vi "TrajectoryParam_calcStuffFwd.vi"(4 "TRAJECTORY_CONFIG":T1={"MaxVelocity"=0.0, "Max Acceleration"=0.0, "StartVelocity"=0.0, "End Velocity"=0.0, "Reversed"=FALSE, "DiffDrKineConstntDefined"=FALSE, "CentAcellConstntDefined"=FALSE, "DiffDrVoltConstntDefined"=FALSE, "DIFF_DRIVE_KINE_CONSTRAINT"={"Max Speed (M/S)"=0.0, "DIFF_DRIVE_KINEMATICS"={"TrackWidth_Meters"=0.0}}, "CENTRIPETAL_ACCEL_CONSTRAINT"={"Max Cent Accel"=0.0}, "SwerveDrKineConstntDefined"=FALSE, "SWERVE_DRIVE_KINE_CONSTRAINT"={"Max Speed (M/S)"=0.0, "SwerveKinematics"={"NumModules"=0, "InverseKinematics"=[], "ForwardKinematics"=[], "Modules"=[], "PrevCoR"={"X"=0.0, "Y"=0.0}}}, "DIFF_DRIVE_VOLTAGE_CONSTRAINT"={"Max Voltage"=0.0, "DIFF_DRIVE_KINEMATICS"={"TrackWidth_Meters"=0.0}, "SIMPLE_MOTOR_FF"={"Ks"=0.0, "Kv"=0.0, "Ka"=0.0}}, "MECANUM_DRIVE_KINE_CONSTRAINT"={"Max Speed (M/S)"=0.0, "MECA_DRIVE_KINEMATICS"={"FrontLeft"={"X"=0.0, "Y"=0.0}, "FrontRight"={"X"=0.0, "Y"=0.0}, "RearLeft"={"X"=0.0, "Y"=0.0}, "RearRight"={"X"=0.0, "Y"=0.0}, "InverseKinematics"=[[0.0, 1.0, -1.0, 0.0], [0.0, 1.0, 1.0, 0.0], [0.0, 1.0, 1.0, 0.0], [0.0, 1.0, -1.0, 0.0]], "ForwardKinematics"=[[0.0, 1.0, -1.0, 0.0], [0.0, 1.0, 1.0, 0.0], [0.0, 1.0, 1.0, 0.0], [0.0, 1.0, -1.0, 0.0]], "PrevCoR"={"X"=0.0, "Y"=0.0}}}, "MecanumDrKineConstntDefined"=FALSE} {"MECANUM_DRIVE_KINE_CONSTRAINT"."MECA_DRIVE_KINEMATICS"."PrevCoR"."Y" format="%14.3f"; "MECANUM_DRIVE_KINE_CONSTRAINT"."MECA_DRIVE_KINEMATICS"."PrevCoR"."X" format="%14.3f"; "MECANUM_DRIVE_KINE_CONSTRAINT"."MECA_DRIVE_KINEMATICS"."RearRight"."Y" format="%14.3f"; "MECANUM_DRIVE_KINE_CONSTRAINT"."MECA_DRIVE_KINEMATICS"."RearRight"."X" format="%14.3f"; "MECANUM_DRIVE_KINE_CONSTRAINT"."MECA_DRIVE_KINEMATICS"."RearLeft"."Y" format="%14.3f"; "MECANUM_DRIVE_KINE_CONSTRAINT"."MECA_DRIVE_KINEMATICS"."RearLeft"."X" format="%14.3f"; "MECANUM_DRIVE_KINE_CONSTRAINT"."MECA_DRIVE_KINEMATICS"."FrontRight"."Y" format="%14.3f"; "MECANUM_DRIVE_KINE_CONSTRAINT"."MECA_DRIVE_KINEMATICS"."FrontRight"."X" format="%14.3f"; "MECANUM_DRIVE_KINE_CONSTRAINT"."MECA_DRIVE_KINEMATICS"."FrontLeft"."Y" format="%14.3f"; "MECANUM_DRIVE_KINE_CONSTRAINT"."MECA_DRIVE_KINEMATICS"."FrontLeft"."X" format="%14.3f"; "MECANUM_DRIVE_KINE_CONSTRAINT"."Max Speed (M/S)" format="%20.4f"; "DIFF_DRIVE_VOLTAGE_CONSTRAINT"."SIMPLE_MOTOR_FF"."Ka" format="%13.4f"; "DIFF_DRIVE_VOLTAGE_CONSTRAINT"."SIMPLE_MOTOR_FF"."Kv" format="%13.4f"; "DIFF_DRIVE_VOLTAGE_CONSTRAINT"."SIMPLE_MOTOR_FF"."Ks" format="%13.4f"; "DIFF_DRIVE_VOLTAGE_CONSTRAINT"."DIFF_DRIVE_KINEMATICS"."TrackWidth_Meters" format="%20.4f"; "DIFF_DRIVE_VOLTAGE_CONSTRAINT"."Max Voltage" format="%20.4f"; "SWERVE_DRIVE_KINE_CONSTRAINT"."SwerveKinematics"."PrevCoR"."Y" format="%14.3f"; "SWERVE_DRIVE_KINE_CONSTRAINT"."SwerveKinematics"."PrevCoR"."X" format="%14.3f"; "SWERVE_DRIVE_KINE_CONSTRAINT"."SwerveKinematics"."Modules"."Y" format="%14.3f"; "SWERVE_DRIVE_KINE_CONSTRAINT"."SwerveKinematics"."Modules"."X" format="%14.3f"; "SWERVE_DRIVE_KINE_CONSTRAINT"."Max Speed (M/S)" format="%20.4f"; "CENTRIPETAL_ACCEL_CONSTRAINT"."Max Cent Accel" format="%20.4f"; "DIFF_DRIVE_KINE_CONSTRAINT"."DIFF_DRIVE_KINEMATICS"."TrackWidth_Meters" format="%20.4f"; "DIFF_DRIVE_KINE_CONSTRAINT"."Max Speed (M/S)" format="%20.4f"; "End Velocity" format="%20.4f"; "StartVelocity" format="%20.4f"; "Max Acceleration" format="%20.4f"; "MaxVelocity" format="%20.4f"}, 6 "MaxVelocity":dbl, 7 "Reversed":bool, 8 "MaxAccel":dbl, 9 "previousCONSTRAINED_STATEin":T13={"POSEwCURVATURE"={"CURVATURE"=0.0, "POSE"={"TRANSLATION"={"X"=0.0, "Y"=0.0}, "ROTATION"={"VALUE"=0.0, "COS"=1.0, "SIN"=0.0}}}, "Distance"=0.0, "minAccel"=0.0, "maxAccel"=0.0, "maxVelocity"=0.0} {"POSEwCURVATURE"."POSE"."ROTATION"."SIN" format="%13.4f"; "POSEwCURVATURE"."POSE"."ROTATION"."COS" format="%13.4f"; "POSEwCURVATURE"."POSE"."ROTATION"."VALUE" format="%13.4f"; "POSEwCURVATURE"."POSE"."TRANSLATION"."Y" format="%14.3f"; "POSEwCURVATURE"."POSE"."TRANSLATION"."X" format="%14.3f"}, 10 "ds":dbl, 11 "thisCONSTRAINED_STATEin":T13={"POSEwCURVATURE"={"CURVATURE"=0.0, "POSE"={"TRANSLATION"={"X"=0.0, "Y"=0.0}, "ROTATION"={"VALUE"=0.0, "COS"=1.0, "SIN"=0.0}}}, "Distance"=0.0, "minAccel"=0.0, "maxAccel"=0.0, "maxVelocity"=0.0} {"POSEwCURVATURE"."POSE"."ROTATION"."SIN" format="%13.4f"; "POSEwCURVATURE"."POSE"."ROTATION"."COS" format="%13.4f"; "POSEwCURVATURE"."POSE"."ROTATION"."VALUE" format="%13.4f"; "POSEwCURVATURE"."POSE"."TRANSLATION"."Y" format="%14.3f"; "POSEwCURVATURE"."POSE"."TRANSLATION"."X" format="%14.3f"}) -> (0 "error out":errorcluster, 1 "previousCONSTRAINED_STATEout":T13={"POSEwCURVATURE"={"CURVATURE"=0.0, "POSE"={"TRANSLATION"={"X"=0.0, "Y"=0.0}, "ROTATION"={"VALUE"=0.0, "COS"=1.0, "SIN"=0.0}}}, "Distance"=0.0, "minAccel"=0.0, "maxAccel"=0.0, "maxVelocity"=0.0} {"POSEwCURVATURE"."POSE"."ROTATION"."SIN" format="%13.4f"; "POSEwCURVATURE"."POSE"."ROTATION"."COS" format="%13.4f"; "POSEwCURVATURE"."POSE"."ROTATION"."VALUE" format="%13.4f"; "POSEwCURVATURE"."POSE"."TRANSLATION"."Y" format="%14.3f"; "POSEwCURVATURE"."POSE"."TRANSLATION"."X" format="%14.3f"}, 3 "thisCONSTRAINED_STATEout":T13={"POSEwCURVATURE"={"CURVATURE"=0.0, "POSE"={"TRANSLATION"={"X"=0.0, "Y"=0.0}, "ROTATION"={"VALUE"=0.0, "COS"=1.0, "SIN"=0.0}}}, "Distance"=0.0, "minAccel"=0.0, "maxAccel"=0.0, "maxVelocity"=0.0} {"POSEwCURVATURE"."POSE"."ROTATION"."SIN" format="%13.4f"; "POSEwCURVATURE"."POSE"."ROTATION"."COS" format="%13.4f"; "POSEwCURVATURE"."POSE"."ROTATION"."VALUE" format="%13.4f"; "POSEwCURVATURE"."POSE"."TRANSLATION"."Y" format="%14.3f"; "POSEwCURVATURE"."POSE"."TRANSLATION"."X" format="%14.3f"})   [LabVIEW 2019, in "Trajectory_Library.lvlib"]
doc: "Internal routine called by TrajectoryParam_timeParam.VI"
uses:
  Trajectory_Library.lvlib
  CONSTRAINED_STATE.ctl
  POSEwCURVATURE.ctl
  POSE2D.ctl
  TRANSLATION2D.ctl
  ROTATION2D.ctl
  TRAJ_CONFIG.ctl
  TRAJ_CONSTRAINT_DIIF_DRIVE_KINEMATICS.ctl
  DIFF_DRIVE_KINEMATICS.ctl
  TRAJ_CONSTRAINT_CENTRIPETAL_ACCEL.ctl
  TRAJ_CONSTRAINT_SWERVE_DRIVE_KINEMATICS.ctl
  SWERVE_DRIVE_KINEMATICS.ctl
  <vilib>/Analysis/Matrix/Datatypes/RealMatrix.ctl
  TRAJ_CONSTRAINT_DIIF_DRIVE_VOLTAGE.ctl
  SIMPLE_MOTOR_FF.ctl
  TRAJ_CONSTRAINT_MECA_DRIVE_KINEMATICS.ctl
  MECA_DRIVE_KINEMATICS.ctl
  <vilib>/Analysis/Matrix/NI_Matrix.lvlib
panel:
  # "ARRAY OF OTHER\nCONSTRAINTS \nGOES HERE.."
  # "All units\nare SI"
  # "All units\nare SI"
  # "All units\nare SI"
  # "All units\nare SI"
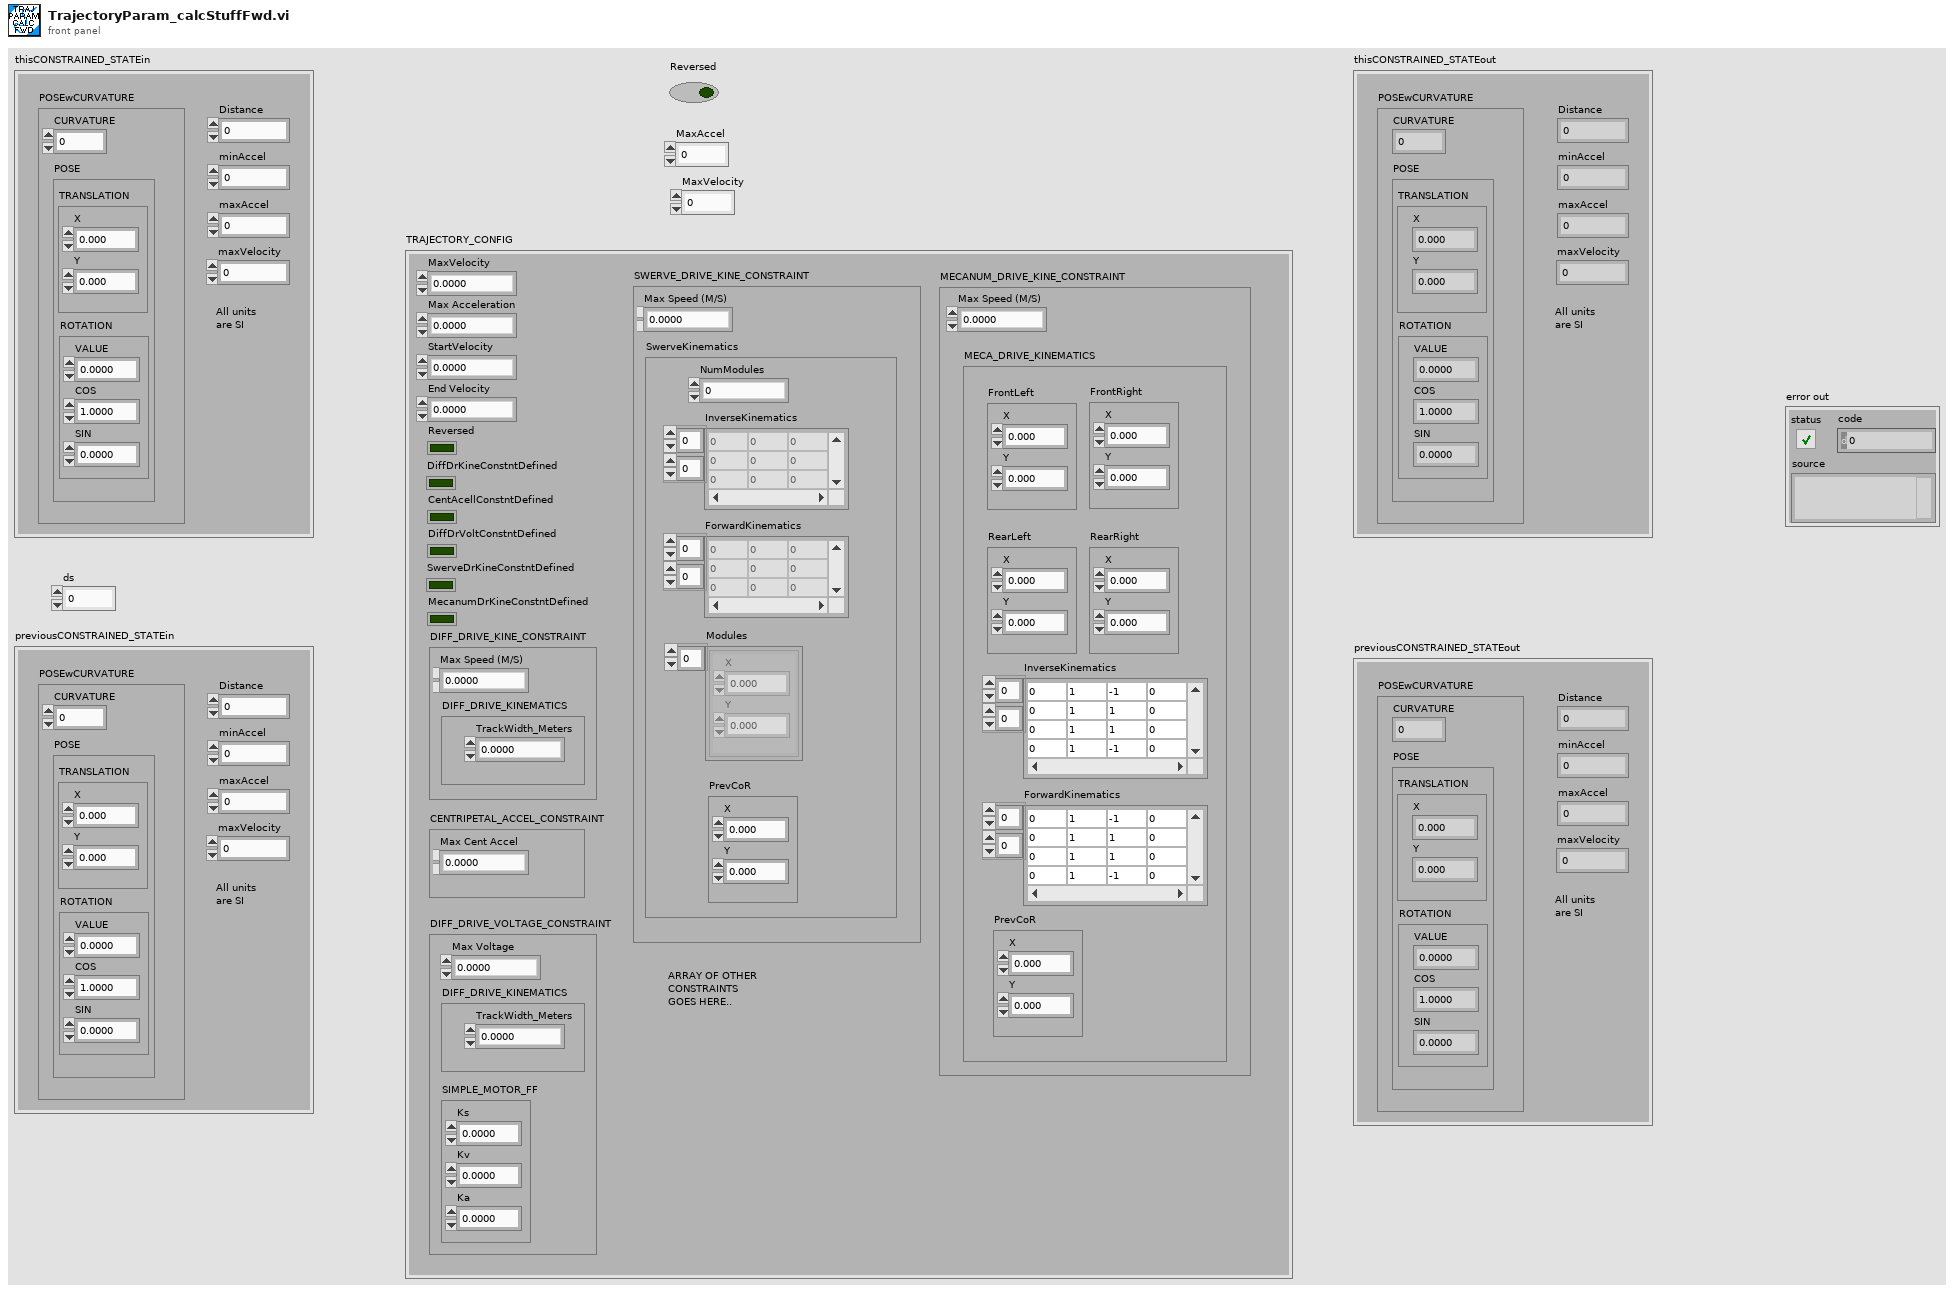
[diagram p1: front panel]
types:
  T1 = typedef "Trajectory_Library.lvlib/TRAJ_CONFIG.ctl" = cluster{"MaxVelocity":dbl, "Max Acceleration":dbl, "StartVelocity":dbl, "End Velocity":dbl, "Reversed":bool, "DiffDrKineConstntDefined":bool, "CentAcellConstntDefined":bool, "DiffDrVoltConstntDefined":bool, "DIFF_DRIVE_KINE_CONSTRAINT":T2, "CENTRIPETAL_ACCEL_CONSTRAINT":T4, "SwerveDrKineConstntDefined":bool, "SWERVE_DRIVE_KINE_CONSTRAINT":T5, "DIFF_DRIVE_VOLTAGE_CONSTRAINT":T9, "MECANUM_DRIVE_KINE_CONSTRAINT":T11, "MecanumDrKineConstntDefined":bool}
  T2 = typedef "Trajectory_Library.lvlib/TRAJ_CONSTRAINT_DIIF_DRIVE_KINEMATICS.ctl" = cluster{"Max Speed (M/S)":dbl, "DIFF_DRIVE_KINEMATICS":T3}
  T3 = typedef "Trajectory_Library.lvlib/DIFF_DRIVE_KINEMATICS.ctl" = cluster{"TrackWidth_Meters":dbl}
  T4 = typedef "Trajectory_Library.lvlib/TRAJ_CONSTRAINT_CENTRIPETAL_ACCEL.ctl" = cluster{"Max Cent Accel":dbl}
  T5 = typedef "Trajectory_Library.lvlib/TRAJ_CONSTRAINT_SWERVE_DRIVE_KINEMATICS.ctl" = cluster{"Max Speed (M/S)":dbl, "SwerveKinematics":T6}
  T6 = typedef "Trajectory_Library.lvlib/SWERVE_DRIVE_KINEMATICS.ctl" = cluster{"NumModules":i32, "InverseKinematics":T7, "ForwardKinematics":T7, "Modules":T8[], "PrevCoR":T8}
  T7 = typedef "NI_Matrix.lvlib/RealMatrix.ctl" = dbl[][]
  T8 = typedef "Trajectory_Library.lvlib/TRANSLATION2D.ctl" = cluster{"X":dbl, "Y":dbl}
  T9 = typedef "Trajectory_Library.lvlib/TRAJ_CONSTRAINT_DIIF_DRIVE_VOLTAGE.ctl" = cluster{"Max Voltage":dbl, "DIFF_DRIVE_KINEMATICS":T3, "SIMPLE_MOTOR_FF":T10}
  T10 = typedef "Trajectory_Library.lvlib/SIMPLE_MOTOR_FF.ctl" = cluster{"Ks":dbl, "Kv":dbl, "Ka":dbl}
  T11 = typedef "Trajectory_Library.lvlib/TRAJ_CONSTRAINT_MECA_DRIVE_KINEMATICS.ctl" = cluster{"Max Speed (M/S)":dbl, "MECA_DRIVE_KINEMATICS":T12}
  T12 = typedef "Trajectory_Library.lvlib/MECA_DRIVE_KINEMATICS.ctl" = cluster{"FrontLeft":T8, "FrontRight":T8, "RearLeft":T8, "RearRight":T8, "InverseKinematics":T7, "ForwardKinematics":T7, "PrevCoR":T8}
  T13 = typedef "Trajectory_Library.lvlib/CONSTRAINED_STATE.ctl" = cluster{"POSEwCURVATURE":T14, "Distance":dbl, "minAccel":dbl, "maxAccel":dbl, "maxVelocity":dbl}
  T14 = typedef "Trajectory_Library.lvlib/POSEwCURVATURE.ctl" = cluster{"CURVATURE":dbl, "POSE":T15}
  T15 = typedef "Trajectory_Library.lvlib/POSE2D.ctl" = cluster{"TRANSLATION":T8, "ROTATION":T16}
  T16 = typedef "Trajectory_Library.lvlib/ROTATION2D.ctl" = cluster{"VALUE":dbl, "COS":dbl, "SIN":dbl}
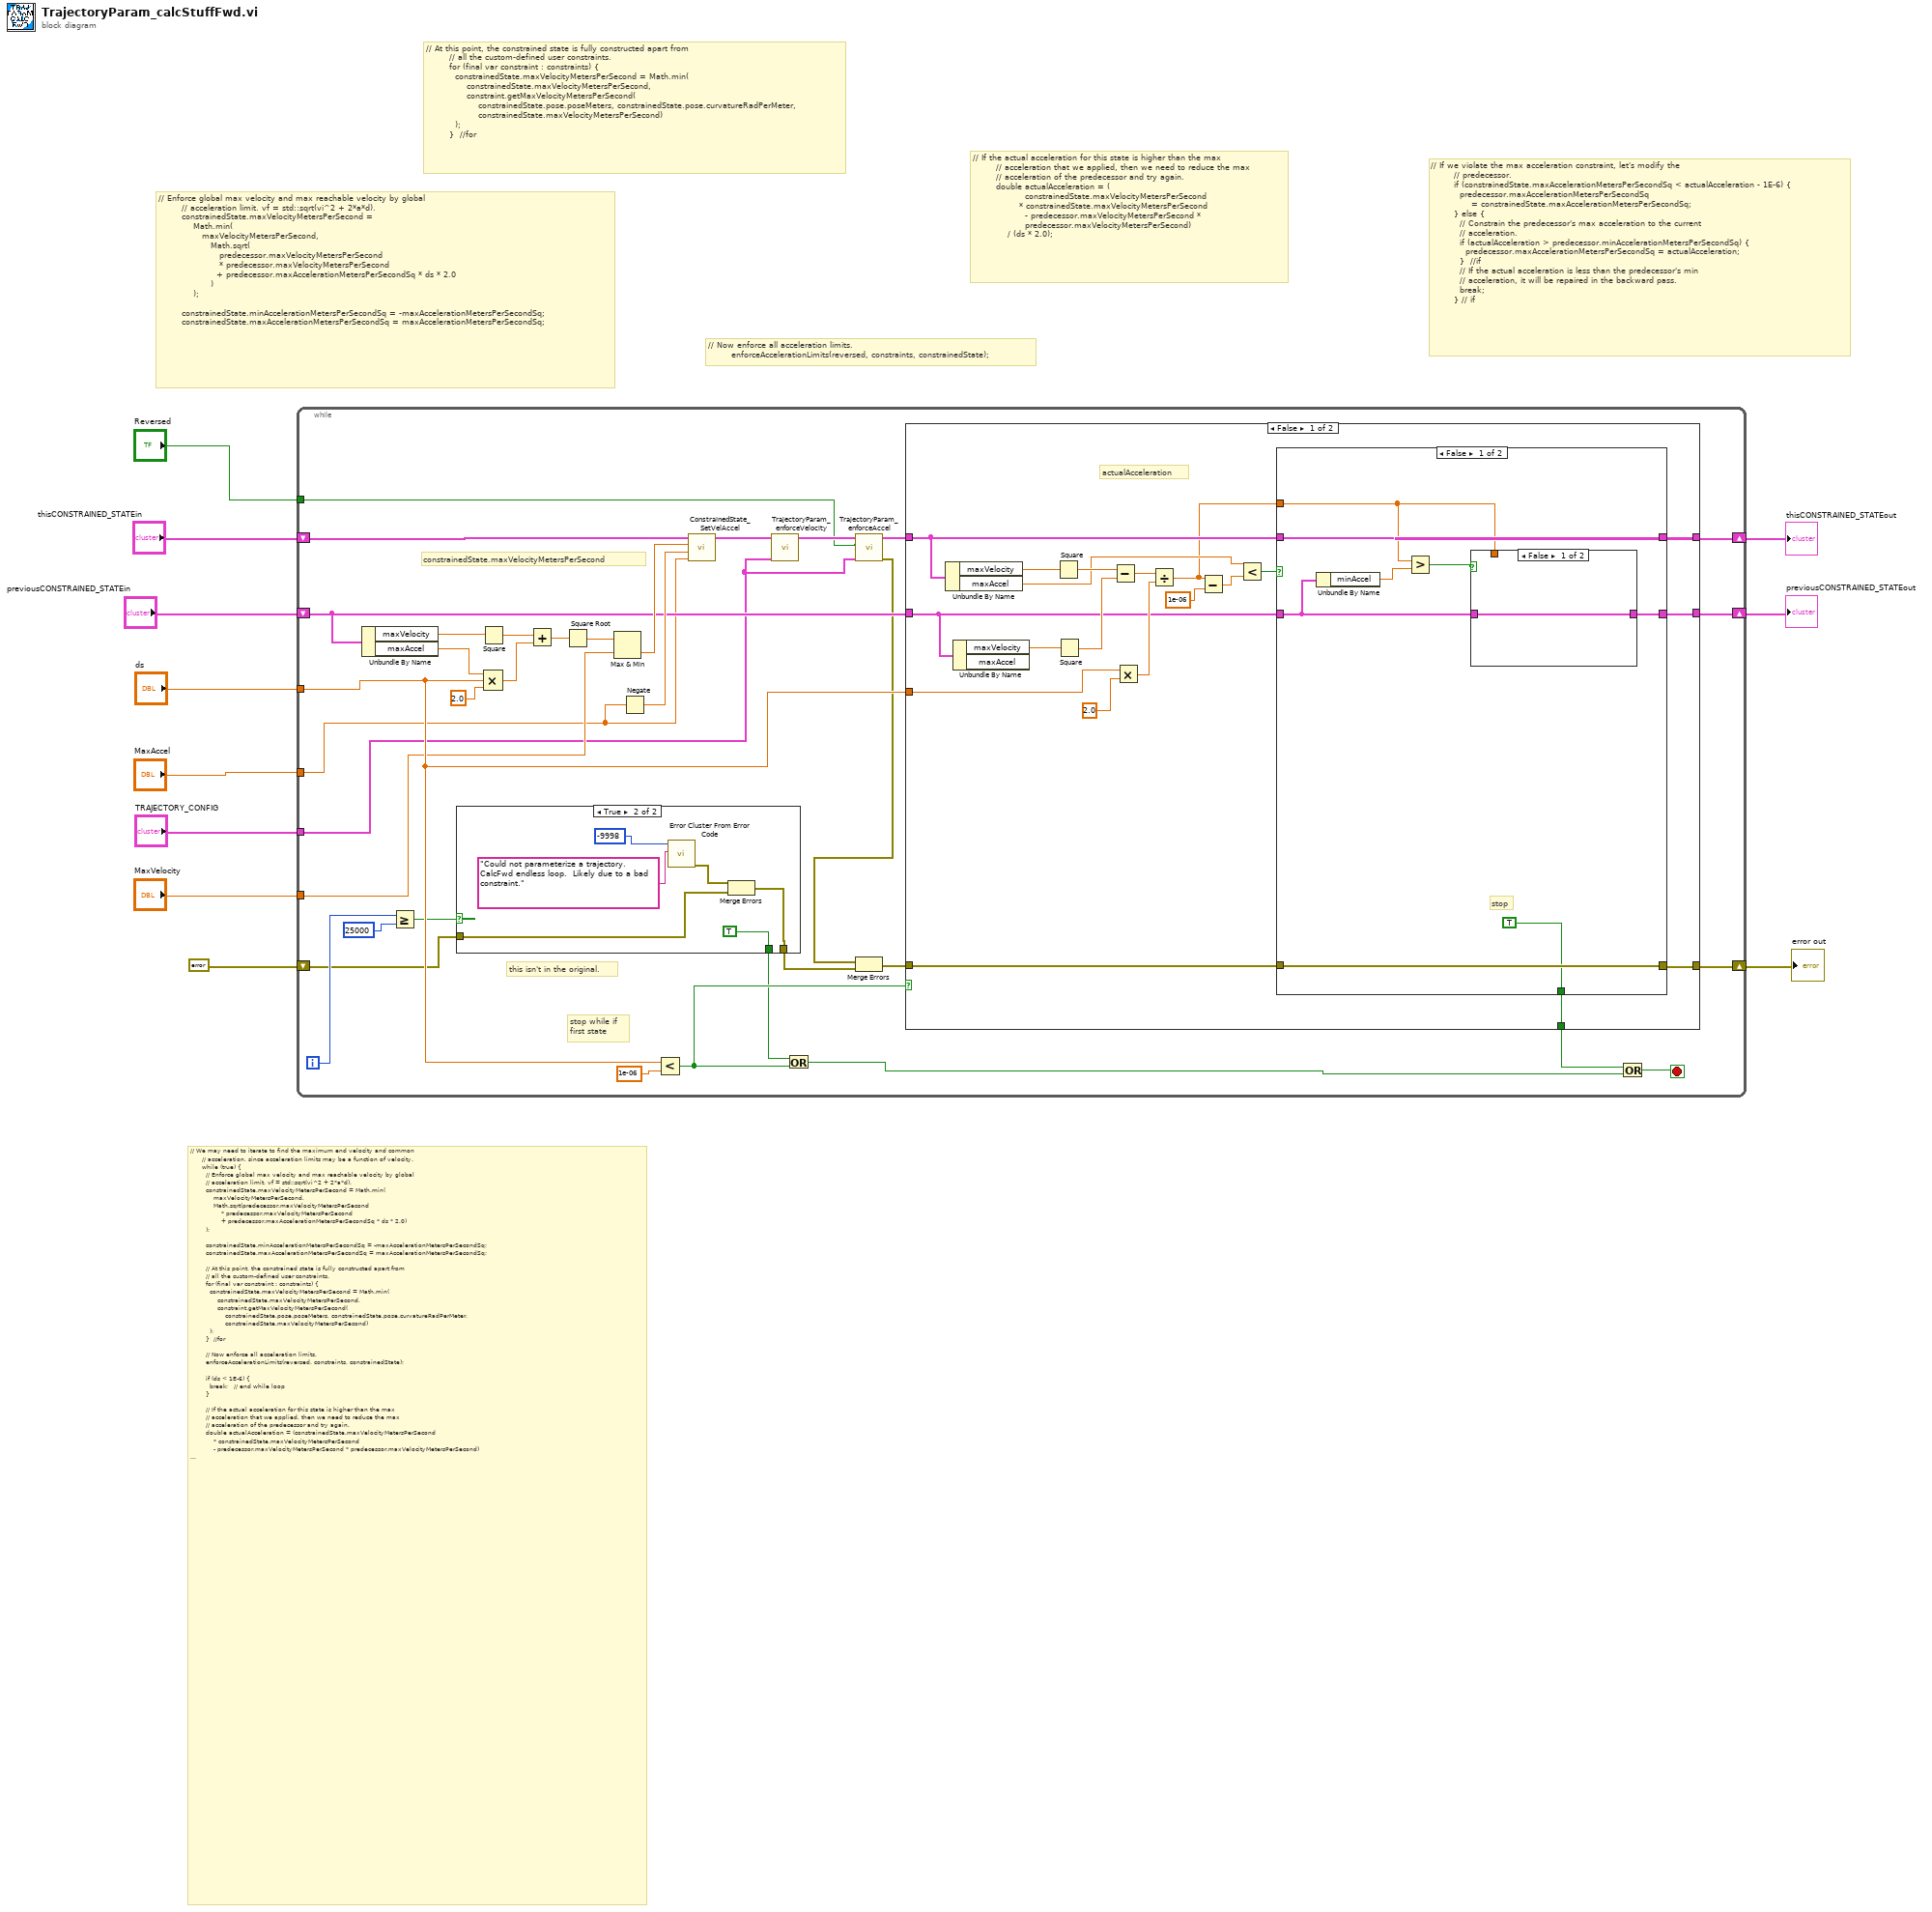
[diagram p0: block diagram]
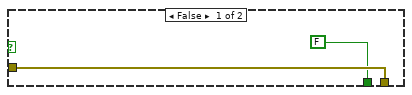
[diagram p2: hidden frame]
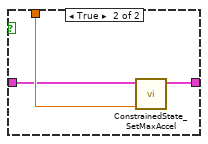
[diagram p3: hidden frame]
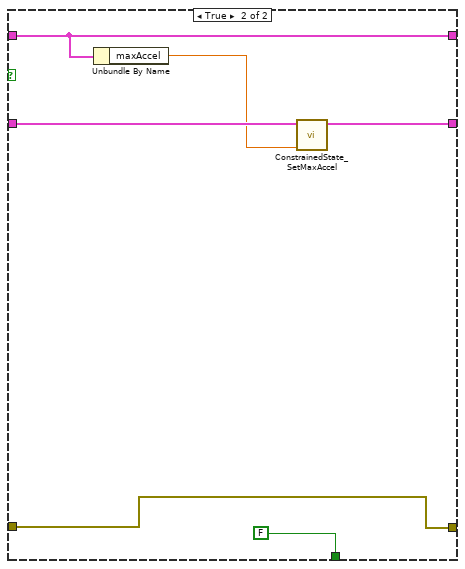
[diagram p4: hidden frame]
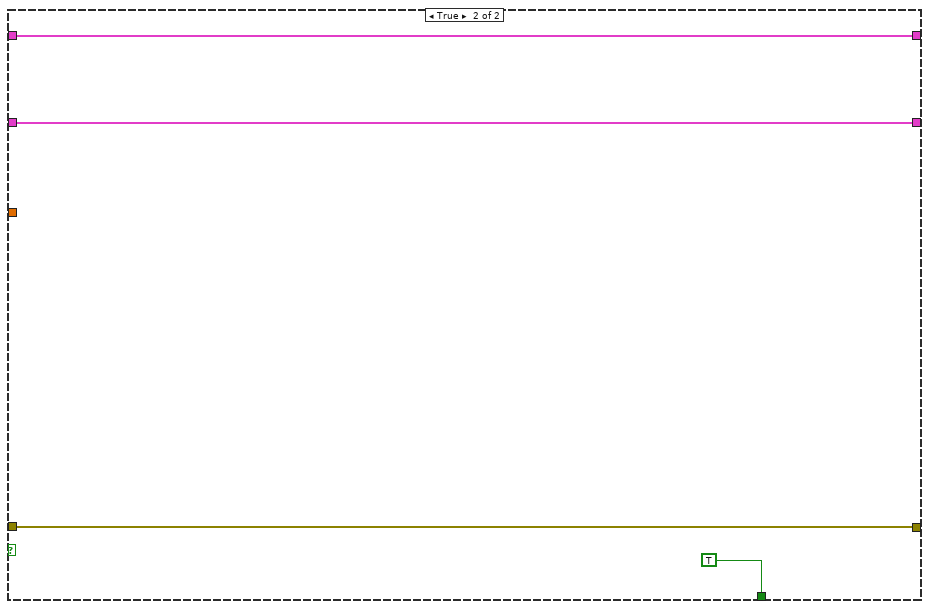
[diagram p5: hidden frame]
diagram:
  # "// If we violate the max acceleration constraint, let's modify the\n        // predecessor.\n        if (constrainedState.maxAccelerationMetersPerSecondSq < actualAcceleration - 1E-6) {\n          predecessor.maxAccelerationMetersPerSecondSq\n              = constrainedState.maxAccelerationMetersPerSecondSq;\n        } else {\n          // Constrain the predecessor's max acceleration to the current\n          // acceleration.\n          if (actualAcceleration > predecessor.minAccelerationMetersPerSecondSq) {\n            predecessor.maxAccelerationMetersPerSecondSq = actualAcceleration;\n          }  //if\n          // If the actual acceleration is less than the predecessor's min\n          // acceleration, it will be repaired in the backward pass.\n          break;\n        } // if"
  # "// If the actual acceleration for this state is higher than the max\n        // acceleration that we applied, then we need to reduce the max\n        // acceleration of the predecessor and try again.\n        double actualAcceleration = (\n                  constrainedState.maxVelocityMetersPerSecond\n                * constrainedState.maxVelocityMetersPerSecond\n                  - predecessor.maxVelocityMetersPerSecond * \n                  predecessor.maxVelocityMetersPerSecond)\n            / (ds * 2.0);"
  # "// Now enforce all acceleration limits.\n        enforceAccelerationLimits(reversed, constraints, constrainedState);"
  # "// At this point, the constrained state is fully constructed apart from\n        // all the custom-defined user constraints.\n        for (final var constraint : constraints) {\n          constrainedState.maxVelocityMetersPerSecond = Math.min(\n              constrainedState.maxVelocityMetersPerSecond,\n              constraint.getMaxVelocityMetersPerSecond(\n                  constrainedState.pose.poseMeters, constrainedState.pose.curvatureRadPerMeter,\n                  constrainedState.maxVelocityMetersPerSecond)\n          );\n        }  //for"
  # "// Enforce global max velocity and max reachable velocity by global\n        // acceleration limit. vf = std::sqrt(vi^2 + 2*a*d).\n        constrainedState.maxVelocityMetersPerSecond = \n            Math.min(\n               maxVelocityMetersPerSecond,\n                  Math.sqrt(\n                     predecessor.maxVelocityMetersPerSecond\n                     * predecessor.maxVelocityMetersPerSecond\n                    + predecessor.maxAccelerationMetersPerSecondSq * ds * 2.0\n                  )\n            ); \n\n        constrainedState.minAccelerationMetersPerSecondSq = -maxAccelerationMetersPerSecondSq;\n        constrainedState.maxAccelerationMetersPerSecondSq = maxAccelerationMetersPerSecondSq;"
  # "// We may need to iterate to find the maximum end velocity and common\n      // acceleration, since acceleration limits may be a function of velocity.\n      while (true) {\n        // Enforce global max velocity and max reachable velocity by global\n        // acceleration limit. vf = std::sqrt(vi^2 + 2*a*d).\n        constrainedState.maxVelocityMetersPerSecond = Math.min(\n            maxVelocityMetersPerSecond,\n            Math.sqrt(predecessor.maxVelocityMetersPerSecond\n                * predecessor.maxVelocityMetersPerSecond\n                + predecessor.maxAccelerationMetersPerSecondSq * ds * 2.0)\n        ); \n\n        constrainedState.minAccelerationMetersPerSecondSq = -maxAccelerationMetersPerSecondSq;\n        constrainedState.maxAccelerationMetersPerSecondSq = maxAccelerationMetersPerSecondSq;\n\n        // At this point, the constrained state is fully constructed apart from\n        // all the custom-defined user constraints.\n        for (final var constraint : constraints) {\n          constrainedState.maxVelocityMetersPerSecond = Math.min(\n              constrainedState.maxVelocityMetersPerSecond,\n              constraint.getMaxVelocityMetersPerSecond(\n                  constrainedState.pose.poseMeters, constrainedState.pose.curvatureRadPerMeter,\n                  constrainedState.maxVelocityMetersPerSecond)\n          );\n        }  //for\n\n        // Now enforce all acceleration limits.\n        enforceAccelerationLimits(reversed, constraints, constrainedState);\n\n        if (ds < 1E-6) {\n          break;   // end while loop\n        }\n\n        // If the actual acceleration for this state is higher than the max\n        // acceleration that we applied, then we need to reduce the max\n        // acceleration of the predecessor and try again.\n        double actualAcceleration = (constrainedState.maxVelocityMetersPerSecond\n            * constrainedState.maxVelocityMetersPerSecond\n            - predecessor.maxVelocityMetersPerSecond * predecessor.maxVelocityMetersPerSecond)\n            / (ds * 2.0);\n\n        // If we violate the max acceleration constraint, let's modify the\n        // predecessor.\n        if (constrainedState.maxAccelerationMetersPerSecondSq < actualAcceleration - 1E-6) {\n          predecessor.maxAccelerationMetersPerSecondSq\n              = constrainedState.maxAccelerationMetersPerSecondSq;\n        } else {\n          // Constrain the predecessor's max acceleration to the current\n          // acceleration.\n          if (actualAcceleration > predecessor.minAccelerationMetersPerSecondSq) {\n            predecessor.maxAccelerationMetersPerSecondSq = actualAcceleration;\n          }  //if\n          // If the actual acceleration is less than the predecessor's min\n          // acceleration, it will be repaired in the backward pass.\n          break;\n        } // if\n      }  // while"
  n1 = while {
    tunnel: "MaxAccel" -> [w12]
    tunnel: "MaxVelocity" -> [w17]
    tunnel: "ds" -> [w31]
    shift-right: [w34] -> w6
    shift-left: "thisCONSTRAINED_STATEin" -> [w39]
    shift-right: [w33] -> w5
    shift-left: "previousCONSTRAINED_STATEin" -> [w35]
    tunnel: "Reversed" -> [w23]
    shift-right: [w26] -> w2
    shift-left: errorcluster {"status"=FALSE, "code"=0, "source"=""} ("error constant") -> [w16]
    tunnel: "TRAJECTORY_CONFIG" -> [w13]
    i -> [w21]
    stop <- w29 stop-if-true
    # "stop while if \nfirst state"
    # "constrainedState.maxVelocityMetersPerSecond"
    # "this isn't in the original."
    n2 = Unbundle By Name(w35) -> ("maxVelocity"=w46:dbl, "maxAccel"=w44:dbl)
    n3 = Greater Or Equal?(x=w21, y=25000) -> (x >= y?=w22:bool)
    n4 = case shown="True" w22 {
      tunnel: w16 -> [w48 w50]
      tunnel: [w48 w49] -> w15
      tunnel: [FALSE TRUE] -> w14
      frame False {
      }
      frame True {
        n5 = call <vilib>:"Error Cluster From Error Code.vi"("error message (\"\")"="Could not parameterize a trajectory.  CalcFwd endless loop.  Likely due to a bad constraint." ("error message (\"\")"), "error code (0)"=-9998) -> ("error out"=w51:errorcluster)  [unwired: 7 in]
        n6 = Merge Errors(w51, w50) -> (w49:errorcluster)
      }
    }
    n7 = Square(x=w46) -> (x^2=w45:dbl)
    n8 = Compound Arithmetic op=MULTIPLY(w44, w31, 2.0 ("value")) -> (w42:dbl)
    n9 = Add(x=w45, y=w42) -> (x+y=w41:dbl)
    n10 = Square Root(x=w41) -> (sqrt(x)=w40:dbl)
    n11 = Max & Min(x=w40, y=w17) -> (min(x,y)=w38:dbl)  [unwired: 1 out]
    n12 = Negate(x=w12) -> (-x=w37:dbl)
    n13 = Less?(x=w31, y=1e-06) -> (x < y?=w19:bool)
    n14 = call "ConstrainedState_SetVelAccel.vi"("maxAcceleration"=w12, "minAcceleration"=w37, "maxVelocity"=w38, "inCONSTRAINED_STATE"=w39) -> ("outCONSTRAINED_STATE"=w25:T13)  [unwired: 7 in]
    n15 = call "TrajectoryParam_enforceVelocity.vi"("TRAJECTORY_CONFIG"=w13, "inCONSTRAINED_STATE"=w25) -> ("outCONSTRAINED_STATE"=w24:T13)  [unwired: 8 in, 1 out]
    n16 = Or(x=w14, y=w19) -> (x .or. y?=w18:bool)
    n17 = call "TrajectoryParam_enforceAccel.vi"("TRAJECTORY_CONFIG"=w13, "Reversed"=w23, "inCONSTRAINED_STATE"=w24) -> ("error out"=w28:errorcluster, "outCONSTRAINED_STATE"=w32:T13)  [unwired: 7 in]
    n18 = Merge Errors(w28, w15) -> (w27:errorcluster)
    n19 = case shown="False" w19 {
      tunnel: w32 -> [w61 w96]
      tunnel: w35 -> [w63 w95]
      tunnel: [w60 w96] -> w34
      tunnel: [w62 w95] -> w33
      tunnel: w31 -> [w70 _]
      tunnel: [w59 TRUE] -> w30
      tunnel: w27 -> [w56 w93]
      tunnel: [w57 w93] -> w26
      frame False {
        # "actualAcceleration"
        n20 = Unbundle By Name(w61) -> ("maxVelocity"=w73:dbl, "maxAccel"=w65:dbl)
        n21 = Unbundle By Name(w63) -> ("maxVelocity"=w74:dbl)  [unwired: 1 out]
        n22 = Square(x=w73) -> (x^2=w72:dbl)
        n23 = Square(x=w74) -> (x^2=w71:dbl)
        n24 = Subtract(x=w72, y=w71) -> (x-y=w69:dbl)
        n25 = Multiply(x=w70, y=2.0) -> (x*y=w68:dbl)
        n26 = Divide(x=w69, y=w68) -> (x/y=w58:dbl)
        n27 = Subtract(x=w58, y=1e-06) -> (x-y=w66:dbl)
        n28 = Less?(x=w65, y=w66) -> (x < y?=w64:bool)
        n29 = case shown="False" w64 {
          tunnel: [w79 w91] -> w62
          tunnel: w63 -> [w80 w92]
          tunnel: w61 -> [w78 w90]
          tunnel: [w78 w90] -> w60
          tunnel: [TRUE FALSE] -> w59
          tunnel: w58 -> [w81 _]
          tunnel: [w77 w87] -> w57
          tunnel: w56 -> [w77 w87]
          frame False {
            # "stop"
            n30 = Unbundle By Name(w80) -> ("minAccel"=w82:dbl)
            n31 = Greater?(x=w81, y=w82) -> (0:w76:bool)
            n32 = case shown="False" w76 {
              tunnel: w81 -> [_ w86]
              tunnel: w80 -> [w83 w85]
              tunnel: [w83 w84] -> w79
              frame False {
              }
              frame True {
                n33 = call "ConstrainedState_SetMaxAccel.vi"("maxAcceleration"=w86, "inCONSTRAINED_STATE"=w85) -> ("outCONSTRAINED_STATE"=w84:T13)  [unwired: 9 in]
              }
            }
          }
          frame True {
            n34 = Unbundle By Name(w90) -> ("maxAccel"=w89:dbl)
            n35 = call "ConstrainedState_SetMaxAccel.vi"("maxAcceleration"=w89, "inCONSTRAINED_STATE"=w92) -> ("outCONSTRAINED_STATE"=w91:T13)  [unwired: 9 in]
          }
        }
      }
      frame True {
      }
    }
    n36 = Or(x=w30, y=w18) -> (x .or. y?=w29:bool)
  }
  "error out" <- w2
  "thisCONSTRAINED_STATEout" <- w6
  "previousCONSTRAINED_STATEout" <- w5
